vi "Update Counters.vi"(7 "当前丢失点":i32, 8 "当前重复点":i32, 9 "生产者迭代":i32, 10 "前一个生产者迭代":i32) -> (0 "更新的丢失点":i32, 1 "更新的重复点":i32)   [LabVIEW 2012]
doc: "本VI根据“生产者循环”的当前迭代计数和前一次迭代计数确定“消费者循环”数据是否丢失或重复。根据数据是否丢失/重复，本VI对丢失/重复计数进行更新。"
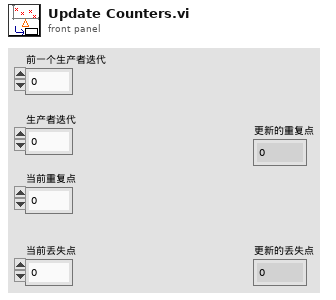
[diagram p1: front panel]
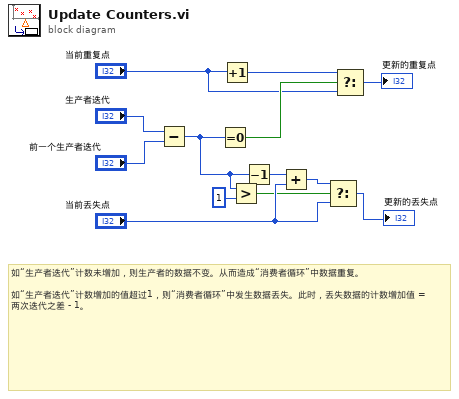
[diagram p0: block diagram]
diagram:
  # "如“生产者迭代”计数未增加，则生产者的数据不变。从而造成“消费者循环”中数据重复。\n\n如“生产者迭代”计数增加的值超过1，则“消费者循环”中发生数据丢失。此时，丢失数据的计数增加值 = 两次迭代之差 - 1。"
  n1 = Subtract ("减")(x="生产者迭代", y="前一个生产者迭代") -> (x-y=w6:i32)
  n2 = Equal To 0? ("等于0？")(x=w6) -> (x = 0?=w9:bool)
  n3 = Increment ("加1")(x="当前重复点") -> (x+1=w8:i32)
  n4 = Greater? ("大于？")(x=w6, y=1) -> (0:w3:bool)
  n5 = Decrement ("减1")(x=w6) -> (x-1=w1:i32)
  n6 = Add ("加")(x=w1, y="当前丢失点") -> (x+y=w5:i32)
  n7 = Select ("选择")(t=w5, s=w3, f="当前丢失点") -> (s? t:f=→"更新的丢失点":i32)
  n8 = Select ("选择")(t=w8, s=w9, f="当前重复点") -> (s? t:f=→"更新的重复点":i32)
